vi "Write JSON File.vi"   [LabVIEW 2015, in "JSON.lvlib"]
uses:
  JSON.lvlib
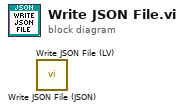
[diagram p0: block diagram]
diagram:
  n1 = call "Write JSON File (JSON).vi"() -> ()  [unwired: 11 in, 1 out]
  n2 = call "Write JSON File (LV).vi"() -> ()  [unwired: 11 in, 1 out]
